vi "___save_2d_data_with_header.vi"(6 "ヘッダー":string, 7 "プロンプト":string, 8 "配列":dbl[][](array[numeric])=[[0.01, 0.02, 0.03, 0.04, 0.05], [0.0013018453356991692, 0.001660848198838855, 0.002691465525605318, 0.0011561349743810848, 0.0011671909844345693]], 9 "形式":string="%^.5e", 10 "file_name":string, 11 "パス":path) -> (3 "出力パス":path)   [LabVIEW 2017]
uses:
  <vilib>/Utility/file.llb/Write To Spreadsheet File (DBL).vi
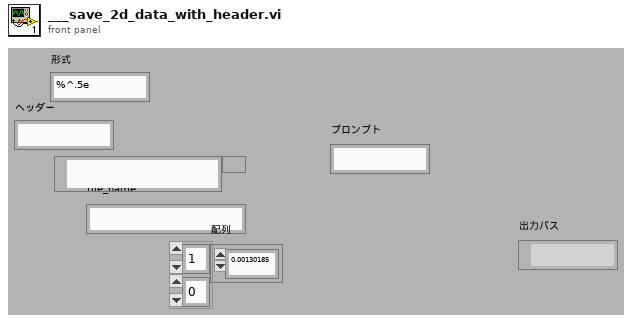
[diagram p1: front panel]
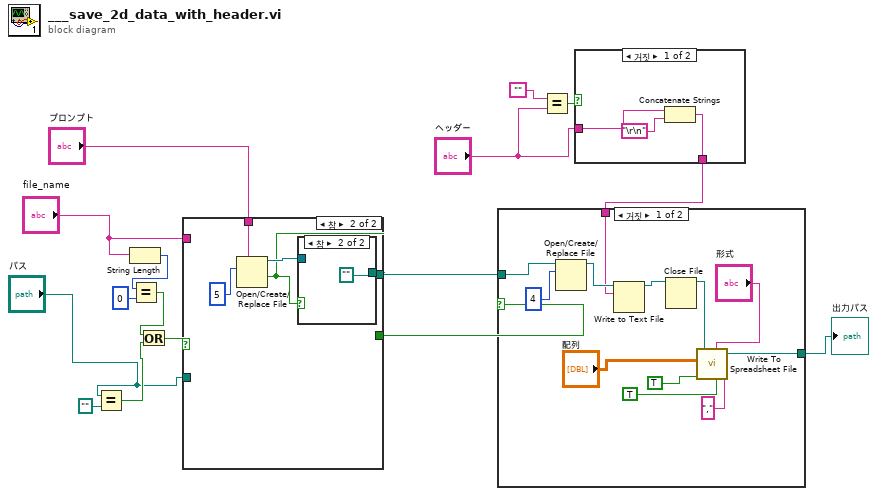
[diagram p0: block diagram]
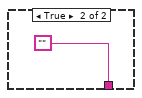
[diagram p2: hidden frame]
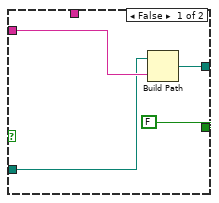
[diagram p4: hidden frame]
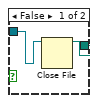
[diagram p5: hidden frame]
diagram:
  n1 = Equal?(x="パス", y=path "") -> (x = y?=w2:bool)
  n2 = String Length(string="file_name") -> (length=w16:i32)
  n3 = Equal?(x=w16, y=0) -> (x = y?=w3:bool)
  n4 = Or(x=w3, y=w2) -> (x .or. y?=w4:bool)
  n5 = case shown="참" w4 {
    tunnel: "file_name" -> [w20 _]
    tunnel: [w19 w23] -> w12
    tunnel: [FALSE w22] -> w13
    tunnel: "プロンプト" -> [_ w21]
    tunnel: "パス" -> [w17 _]
    frame False {
      n6 = Build Path(base path=w17, name or relative path=w20) -> (appended path=w19:path)
    }
    frame True {
      n7 = Open/Create/Replace File(prompt=w21, operation (0:open)=5) -> (refnum out=w24:refnum<file>, cancelled=w22:bool)  [unwired: 4 in, 1 out]
      n8 = case shown="참" w22 {
        tunnel: w24 -> [w27 _]
        tunnel: [w26 path ""] -> w23
        frame False {
          n9 = Close File(refnum=w27) -> (path=w26:path)  [unwired: 1 in, 1 out]
        }
        frame True {
        }
      }
    }
  }
  n10 = Equal?(x="", y="ヘッダー") -> (x = y?=w8:bool)
  n11 = case shown="거짓" w8 {
    tunnel: "ヘッダー" -> [w30 _]
    tunnel: [w29 ""] -> w6
    frame False {
      n12 = Concatenate Strings(w30, "\r\n") -> (w29:string)
    }
    frame True {
    }
  }
  n13 = case shown="거짓" w13 {
    tunnel: w12 -> [w42 w45]
    tunnel: w6 -> [w39 _]
    tunnel: [w33 w45] -> w10
    frame False {
      n14 = Open/Create/Replace File(file path (use dialog)=w42, operation (0:open)=4) -> (refnum out=w40:refnum<file>)  [unwired: 4 in, 2 out]
      n15 = Write to Text File(file (use dialog)=w40, text=w39) -> (refnum out=w38:refnum<file>)  [unwired: 2 in, 2 out]
      n16 = Close File(refnum=w38) -> (path=w37:path)  [unwired: 1 in, 1 out]
      n17 = call-poly <vilib>:"Write To Spreadsheet File.vi"("delimiter (\\t)"=",", "transpose? (no:F)"=TRUE, "format (%.3f)"="形式", "append to file? (new file:F)"=TRUE, "2D data"="配列", "file path (dialog if empty)"=w37) -> ("new file path (Not A Path if cancelled)"=w33:path)  [unwired: 2 in]
    }
    frame True {
    }
  }
  "出力パス" <- w10
